vi "TalonSRXConfigMotionMagic.vi"(0 "Device Reference (in)":T1, 1 "Gear Ratio":dbl=1.0, 5 "Cruise Velocity (deg/s)":dbl, 7 "Acceleration (deg/s^2)":dbl, 9 "S-Curve Strength":dbl, 11 "Error (in)":errorcluster) -> (4 "Device Reference (out)":T1, 15 "Error (out)":errorcluster)   [LabVIEW 2020]
doc: "Wrapper function for configuring the Motion Magic parameters for Talon SRX motor controllers."
uses:
  6896a119-edcc-46ad-8f5b-8706f7426cba.vi
  <vilib>/Rock Robotics/SystemInterfaces/DIO/FPGA_DIOPWMChannel.ctl
  <vilib>/Rock Robotics/WPI/PWM/WPI_PWMDeadband.ctl
  <vilib>/Rock Robotics/WPI/MotorControl/WPI_MotorControlType.ctl
  <vilib>/Rock Robotics/SystemInterfaces/DIO/FPGA_DIOChannel.ctl
  <vilib>/Rock Robotics/WPI/MotorControl/WPI_MotorControlDeviceRef.ctl
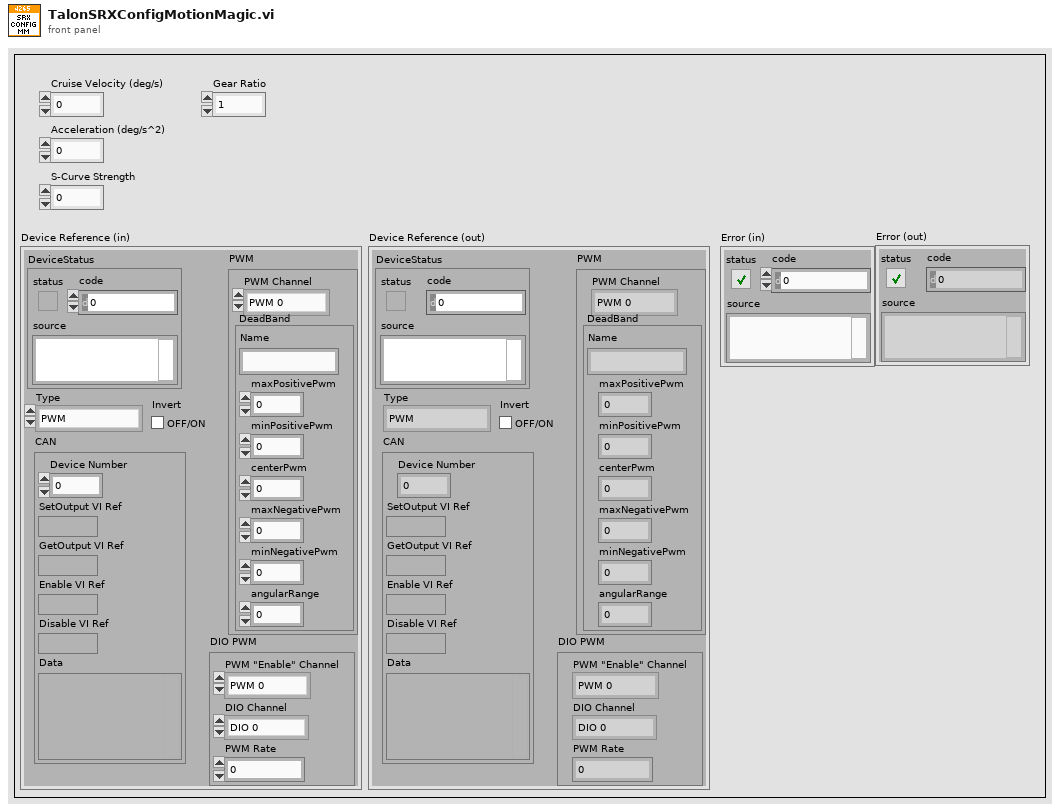
[diagram p1: front panel]
types:
  T1 = typedef "WPI_MotorControlDeviceRef.ctl" = cluster{"DeviceStatus":errorcluster, "Type":T2, "PWM":cluster{"PWM Channel":T3, "DeadBand":T4}, "CAN":cluster{"Device Number":u8, "SetOutput VI Ref":variant, "GetOutput VI Ref":variant, "Enable VI Ref":variant, "Disable VI Ref":variant, "Data":variant}, "Invert":bool, "DIO PWM":cluster{"PWM \"Enable\" Channel":T3, "DIOChannel":T5, "PWM Rate":dbl}}
  T2 = typedef "WPI_MotorControlType.ctl" = enum16{"PWM", "CAN", "DIO PWM"}
  T3 = typedef "FPGA_DIOPWMChannel.ctl" = enum8{"PWM 0", "PWM 1", "PWM 2", "PWM 3", "PWM 4", "PWM 5", "PWM 6", "PWM 7", "PWM 8", "PWM 9", "PWM MXP 0", "PWM MXP 1", "PWM MXP 2", "PWM MXP 3", "PWM MXP 4", "PWM MXP 5", "PWM MXP 6", "PWM MXP 7", "PWM MXP 8", "PWM MXP 9", "Invalid"}
  T4 = typedef "WPI_PWMDeadband.ctl" = cluster{"Name":string, "maxPositivePwm":i32, "minPositivePwm":i32, "centerPwm":i32, "maxNegativePwm":i32, "minNegativePwm":i32, "angularRange":u16}
  T5 = typedef "FPGA_DIOChannel.ctl" = enum8{"DIO 0", "DIO 1", "DIO 2", "DIO 3", "DIO 4", "DIO 5", "DIO 6", "DIO 7", "DIO 8", "DIO 9", "DIO MXP 0", "DIO MXP 1", "DIO MXP 2", "DIO MXP 3", "DIO MXP 4", "DIO MXP 5", "DIO MXP 6", "DIO MXP 7", "DIO MXP 8", "DIO MXP 9", "DIO MXP 10", "DIO MXP 11", "DIO MXP 12", "DIO MXP 13", "DIO MXP 14", "DIO MXP 15", "SPI Port CS1", "SPI Port CS2", "SPI Port CS3", "SPI Port MISO", "SPI Port MOSI", "Invalid"}
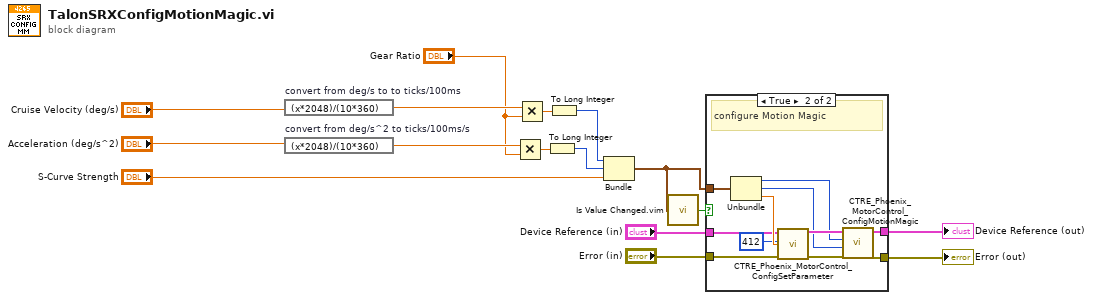
[diagram p0: block diagram]
diagram:
  n1 = expression code="(x*2048)/(10*360)" "convert from deg/s to to ticks/100ms"("Cruise Velocity (deg/s)") -> (w14:dbl)
  n2 = expression code="(x*2048)/(10*360)" "convert from deg/s^2 to ticks/100ms/s"("Acceleration (deg/s^2)") -> (w15:dbl)
  n3 = Multiply(x=w15, y="Gear Ratio") -> (x*y=w4:dbl)
  n4 = Multiply(x=w14, y="Gear Ratio") -> (x*y=w3:dbl)
  n5 = To Long Integer(number=w4) -> (32bit integer=w6:i32)
  n6 = To Long Integer(number=w3) -> (32bit integer=w5:i32)
  n7 = Bundle(w5, w6, "S-Curve Strength"="S-Curve Strength") -> (w7:cluster{i32, i32, "S-Curve Strength":dbl})  [unwired: 1 in]
  n8 = call "Is Value Changed.vim"("value"=w7) -> ("changed or first call?"=w8:bool)
  n9 = case shown="True" w8 {
    tunnel: w7 -> [_ w27]
    tunnel: "Device Reference (in)" -> [w18 w23]
    tunnel: "Error (in)" -> [w17 w22]
    tunnel: [w18 w21] -> w1
    tunnel: [w17 w20] -> w2
    frame False {
    }
    frame True {
      # "configure Motion Magic"
      n10 = Unbundle(w27) -> (w24:i32, w25:i32, "S-Curve Strength"=w26:dbl)
      n11 = call <vilib>:"CTRE_Phoenix_MotorControl_ConfigSetParameter.vi"("PhoenixMotorControlDevRef"=w23, "Parameter"=u16 412, "value"=w26, "error in (no error)"=w22) -> ("PhoenixMotorControlDevRef"=w29:T1, "error out"=w28:errorcluster)  [unwired: 10 in]
      n12 = call <vilib>:"CTRE_Phoenix_MotorControl_ConfigMotionMagic.vi"("error in (no error)"=w28, "Acceleration"=w25, "Cruise Velocity"=w24, "PhoenixMotorControlDevRef"=w29) -> ("error out"=w20:errorcluster, "PhoenixMotorControlDevRef"=w21:T1)  [unwired: 6 in]
    }
  }
  "Error (out)" <- w2
  "Device Reference (out)" <- w1
